vi "SR400 monitoring.vi"(10 "?":bool, 11 "?":bool) -> ()   [LabVIEW 2015]
uses:
  Libraries/SR400/Public/Typedefs/Counter.ctl
  Libraries/SR400/SR400.lvlib
panel:
  in  "Path":path=path "C:/Users/resolution/Desktop/NV_measurements/test/monitoring"
  in  "Count Time Set":dbl[unit]=0.01
  in  "VISA resource name":refnum<visa-resource-name>="GPIB0::18::INSTR"
  out "Counts":dbl=46900.0 format="%#_6e"
  out "Count plot":dbl(graph)=46900.0
  # "Saturate @\n3E+7 c/s"
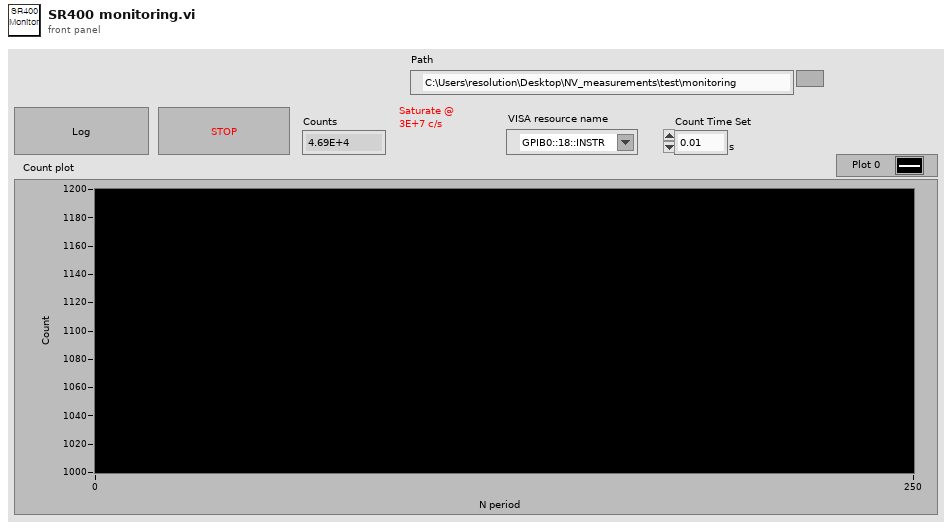
[diagram p1: front panel]
types:
  T1 = enum16{"open", "replace", "create", "open or create", "replace or create", "replace or create with confirmation"}
  T2 = typedef "SR400.lvlib/Counter.ctl" = enum16{"Counter A", "Counter B", "Counter T"}
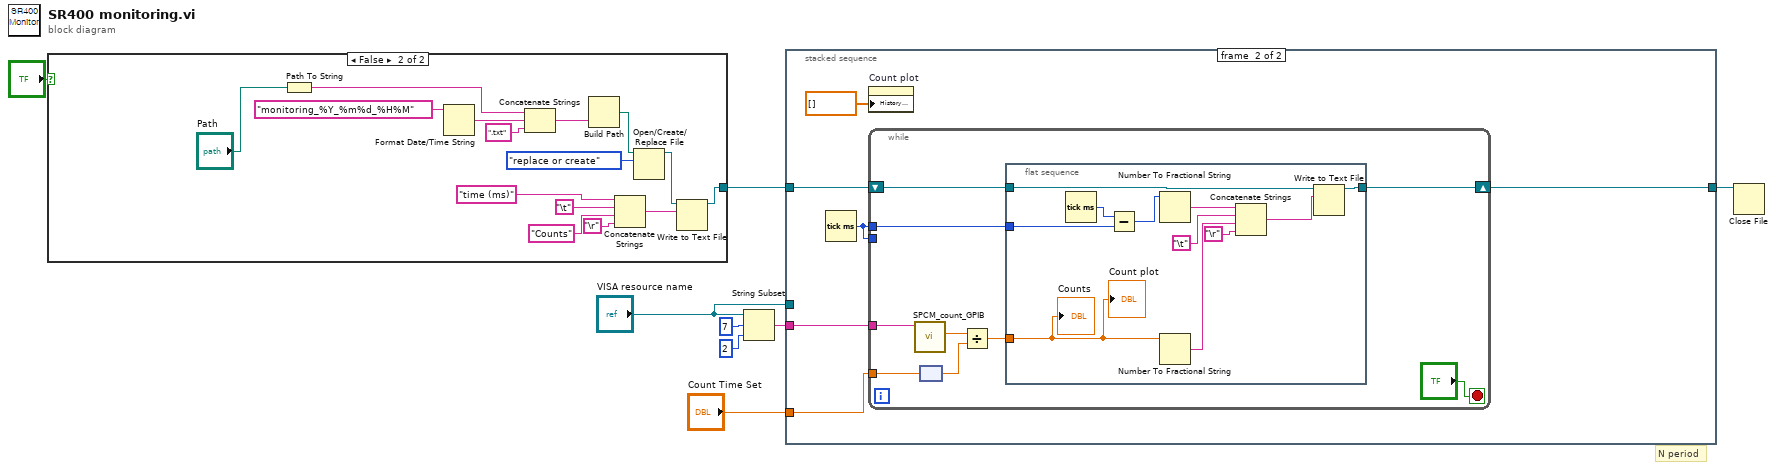
[diagram p0: block diagram]
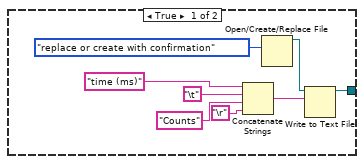
[diagram p2: hidden frame]
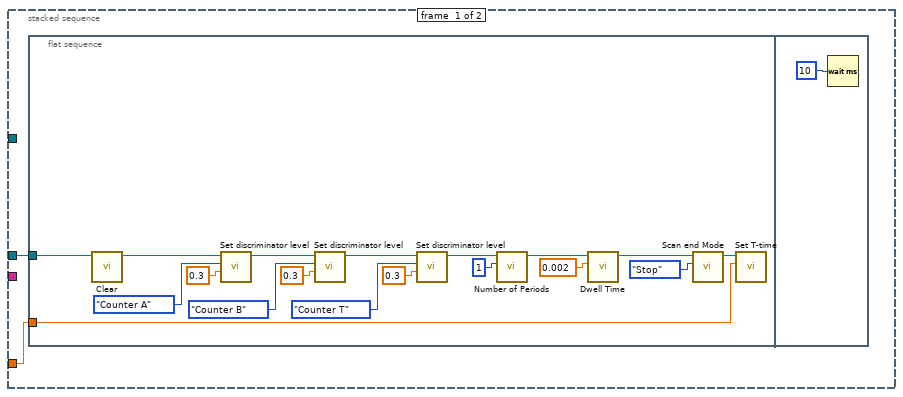
[diagram p3: hidden frame]
diagram:
  # "N period"
  n1 = case shown="False" "?" {
    tunnel: [w9 w24] -> w7
    frame True {
      n2 = Concatenate Strings("time (ms)" ("string"), "\t", "Counts" ("string"), "\r") -> (w15:string)
      n3 = Open/Create/Replace File(operation (0:open)=T1."replace or create with confirmation") -> (refnum out=w16:refnum<file>)  [unwired: 5 in, 2 out]
      n4 = Write to Text File(file (use dialog)=w16, text=w15) -> (refnum out=w9:refnum<file>)  [unwired: 2 in, 2 out]
    }
    frame False {
      n5 = Path To String(path="Path") -> (string=w17:string)
      n6 = Format Date/Time String(time format string (%c)="monitoring_%Y_%m%d_%H%M") -> (date/time string=w29:string)  [unwired: 2 in]
      n7 = Concatenate Strings(w17, w29, ".txt" ("string")) -> (w28:string)
      n8 = Build Path(name or relative path=w28) -> (appended path=w31:path)  [unwired: 1 in]
      n9 = Concatenate Strings("time (ms)" ("string"), "\t", "Counts" ("string"), "\r") -> (w19:string)
      n10 = Open/Create/Replace File(file path (use dialog)=w31, operation (0:open)=T1."replace or create") -> (refnum out=w25:refnum<file>)  [unwired: 4 in, 2 out]
      n11 = Write to Text File(file (use dialog)=w25, text=w19) -> (refnum out=w24:refnum<file>)  [unwired: 2 in, 2 out]
    }
  }
  n12 = String Subset(string="VISA resource name", offset (0)=7, length (rest)=2 ("length (rest)")) -> (substring=w2:string)
  n13 = stacked-sequence {
    tunnel: w2 -> [_ w58]
    tunnel: w7 -> [_ w56]
    tunnel: [_ w55] -> w6
    tunnel: "VISA resource name" -> [w33 _]
    tunnel: "Count Time Set" -> [w32 w53]
    frame #0 {
      n14 = flat-sequence {
        tunnel: w33 -> [w36]
        tunnel: w32 -> [w34]
        frame #0 {
          n15 = call "Clear.vi"("VISA resource name"=w36) -> ("VISA resource name out"=w51:refnum<visa-resource-name>)  [unwired: 9 in, 1 out]
          n16 = call "Set discriminator level.vi"("Level (-0.034 V)"=0.3, "Discriminator (def: A)"=Counter."Counter A", "VISA resource name"=w51) -> ("VISA resource name out"=w48:refnum<visa-resource-name>)  [unwired: 7 in, 1 out]
          n17 = call "Set discriminator level.vi"("Level (-0.034 V)"=0.3, "Discriminator (def: A)"=Counter."Counter B", "VISA resource name"=w48) -> ("VISA resource name out"=w45:refnum<visa-resource-name>)  [unwired: 7 in, 1 out]
          n18 = call "Set discriminator level.vi"("Level (-0.034 V)"=0.3, "Discriminator (def: A)"=Counter."Counter T", "VISA resource name"=w45) -> ("VISA resource name out"=w42:refnum<visa-resource-name>)  [unwired: 7 in, 1 out]
          n19 = call "Number of Periods.vi"("# of periods (def: 1)"=1, "VISA resource name"=w42) -> ("VISA resource name out"=w40:refnum<visa-resource-name>)  [unwired: 8 in, 1 out]
          n20 = call "Dwell Time.vi"("Dwell time (0.002 s)"=0.002, "VISA resource name"=w40) -> ("VISA resource name out"=w38:refnum<visa-resource-name>)  [unwired: 8 in, 1 out]
          n21 = call "Scan end Mode.vi"("Scan End Mode (Def: Stop)"=enum16{"Stop", "Start"}."Stop", "VISA resource name"=w38) -> ("VISA resource name out"=w35:refnum<visa-resource-name>)  [unwired: 8 in, 1 out]
          n22 = call "Set T-time.vi"("Count Time Set"=w34, "VISA resource name"=w35) -> ()  [unwired: 5 in, 3 out]
        }
        frame #1 {
          n23 = Wait (ms)(milliseconds to wait=u32 10) -> ()  [unwired: 1 out]
        }
      }
    }
    frame #1 {
      n24 = Tick Count (ms)() -> (millisecond timer value=w54:u32)
      n25 = property on="Count plot" class="WFChart (strict)"("History Data"=dbl[] []) -> ()  [unwired: 2 in, 2 out]
      n26 = while {
        tunnel: w58 -> [w67]
        tunnel: w54 -> [_]
        tunnel: w54 -> [w65]
        shift-right: [w64] -> w55
        shift-left: w56 -> [w66]
        tunnel: w53 -> [w61]
        stop <- "?" stop-if-true
        n27 = call "SPCM_count_GPIB.vi"("SR400 GPIB Address"=w67) -> ("Counts"=w62:dbl)  [unwired: 10 in]
        n28 = node(w61) -> (w60:dbl)
        n29 = Divide(x=w62, y=w60) -> (x/y=w59:dbl)
        n30 = flat-sequence {
          tunnel: w59 -> [w68]
          tunnel: w66 -> [w70]
          tunnel: w65 -> [w77]
          tunnel: [w69] -> w64
          frame #0 {
            n31 = Tick Count (ms)() -> (millisecond timer value=w78:u32)
            n32 = Subtract(x=w78, y=w77) -> (x-y=w74:u32)
            n33 = Number To Fractional String(number=w74) -> (F-format string=w73:string)  [unwired: 3 in]
            n34 = Number To Fractional String(number=w68) -> (F-format string=w72:string)  [unwired: 3 in]
            n35 = Concatenate Strings(w73, "\t", w72, "\r") -> (w71:string)
            n36 = Write to Text File(file (use dialog)=w70, text=w71) -> (refnum out=w69:refnum<file>)  [unwired: 2 in, 2 out]
            "Count plot" <- w68
            "Counts" <- w68
          }
        }
      }
    }
  }
  n37 = Close File(refnum=w6) -> ()  [unwired: 1 in, 2 out]
